vi "Meas Create Samples Stream MAT File.vi"(7 "data type":T1, 8 "error in":errorcluster, 9 "samples count":i32, 10 "channels count":i32, 11 "binary data file path":path) -> (0 "error out":errorcluster, 3 "stream session":T2)   [LabVIEW 2018]
doc: "Creates MAT file and prepares header for streaming of the sample data. Stream session is returned. When writting is done the variable must be closed. Then next variable can be written."
uses:
  Meas Samples Stream.ctl
  octave/mat/MAT Type Representation.ctl
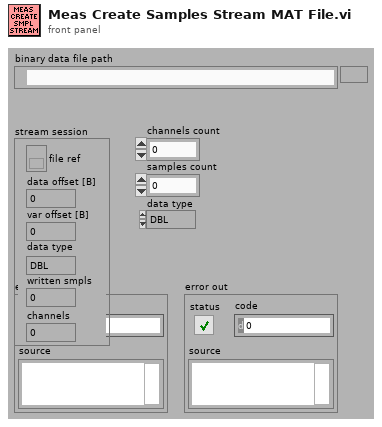
[diagram p1: front panel]
types:
  T1 = typedef "MAT Type Representation.ctl" = enum16{"DBL", "SGL", "I32", "I16", "U16", "U8", "CDB", "CSG", "STR"}
  T2 = typedef "Meas Samples Stream.ctl" = cluster{"file ref":refnum<file>, "data offset [B]":i64, "var offset [B]":i64, "data type":T1, "written smpls":i64, "channels":i64}
  T3 = enum16{"open", "replace", "create", "open or create", "replace or create", "replace or create with confirmation"}
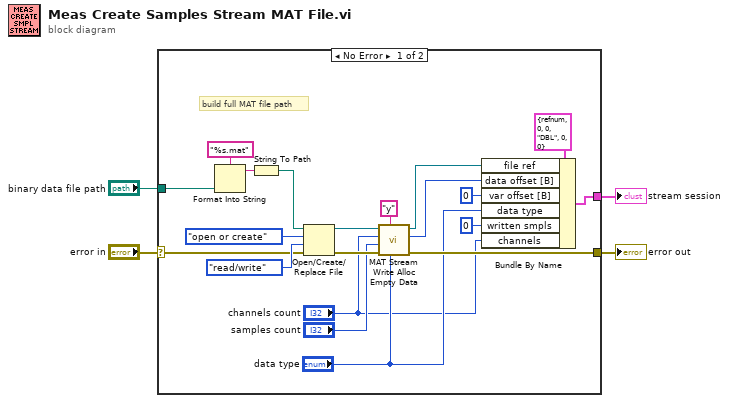
[diagram p0: block diagram]
diagram:
  n1 = case shown="No Error" "error in" {
    selector: "error in" -> [w7 w25]
    tunnel: "binary data file path" -> [w23 _]
    tunnel: [w12 _] -> w3
    tunnel: [w11 w25] -> w2
    frame No Error {
      # "build full MAT file path"
      n2 = Format Into String(format string="%s.mat", w23) -> (resulting string=w21:string)  [unwired: 2 in, 1 out]
      n3 = String To Path(string=w21) -> (path=w20:path)
      n4 = Open/Create/Replace File(file path (use dialog)=w20, error in=w7, operation (0:open)=T3."open or create", access (0:read/write)=enum16{"read/write", "read-only", "write-only"}."read/write") -> (refnum out=w19:refnum<file>, error out=w24:errorcluster)  [unwired: 2 in, 1 out]
      n5 = call "MAT Stream Write Alloc Empty Data.vi"("data type"="data type", "Matrix Name"="y", "error in (no error)"=w24, "columns count"="samples count", "rows count"="channels count", "Ref Num"=w19) -> ("error out"=w11:errorcluster, "data offset [B]"=w13:i64, "Dup Ref Num"=w14:refnum<file>)  [unwired: 2 in, 1 out]
      n6 = Bundle By Name(cluster=T2 {"file ref"=refnum, "data offset [B]"=0, "var offset [B]"=0, "data type"=enum."DBL", "written smpls"=0, "channels"=0} ("stream session"), "file ref"=w14, "data offset [B]"=w13, "var offset [B]"=i64 0, "data type"="data type", "written smpls"=i64 0, "channels"="channels count") -> (w12:T2)
    }
    frame Error {
    }
  }
  "error out" <- w2
  "stream session" <- w3
